vi "StripP(t).vi"(5 "d (depth of curvature)":dbl format="%.2f", 6 "strip (cm)":cluster{"radius":dbl, "h":dbl, "w":dbl}={"radius"=10.0, "h"=5.0, "w"=4.0} {"radius" format="%.2f"; "w" format="%.2f"; "h" format="%.2f"}, 7 "Ring":u16(ring) items=["Strip", "sphere section"], 8 "edge points":dbl[][](array[numeric]) format="%.2f", 9 "waveform sampling rate s":dbl=1e-08 format="%.2e", 10 "drive signal":dbl[](array[numeric])=[-0.5634920634920635, -0.6825396825396826, -0.8015873015873016, -0.9920634920634921, -1.1507936507936507, -1.3888888888888888, -1.992063492063492, -4.2063492063492065, -5.888888888888889, 13.023809523809524, 61.32539682539682, 92.83333333333333, 75.10317460317461, 18.126984126984127, -54.93650793650794, -109.60317460317461, -104.22222222222223, 18.134920634920636, 83.33333333333333, 27.27777777777778, -42.19047619047619, -45.63492063492063, 10.15079365079365, 49.05555555555556, 28.19047619047619, -5.658730158730159, -15.261904761904763, -4.4603174603174605, 7.984126984126984, 10.682539682539682, 5.809523809523809, -0.03968253968253968, -2.515873015873016, -1.4841269841269842, 1.0396825396825398, 2.0555555555555554, 0.9523809523809523, -0.6031746031746031, -1.007936507936508, -0.3968253968253968, 0.14285714285714285] format="%.2f", 11 "P (cm)":cluster{"x":dbl, "y":dbl, "z":dbl}={"x"=-4.0, "y"=0.0, "z"=4.0} {"x" format="%.2f"; "z" format="%.2f"; "y" format="%.2f"}) -> (2 "Waveform Graph":dbl[](graph), 3 "min time shift":dbl format="%.2f")   [LabVIEW 2022 SP3]
panel:
  out "In focal Zone?":bool
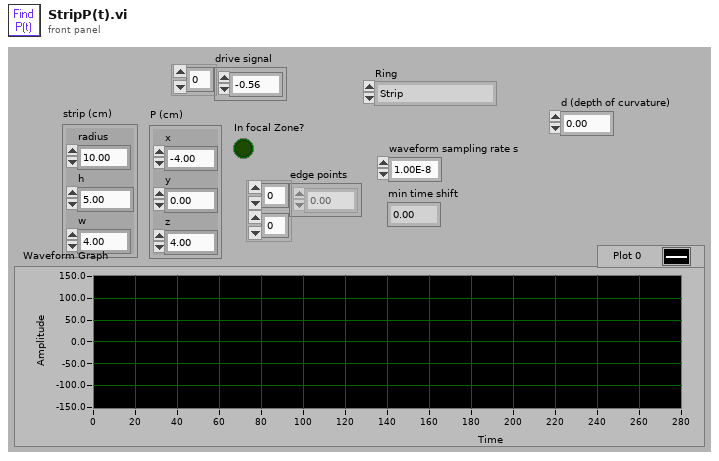
[diagram p1: front panel]
types:
  T1 = cluster{"r":dbl, "d":dbl, "c (cm/s)":dbl, "waveform sampling rate s":dbl, bool}
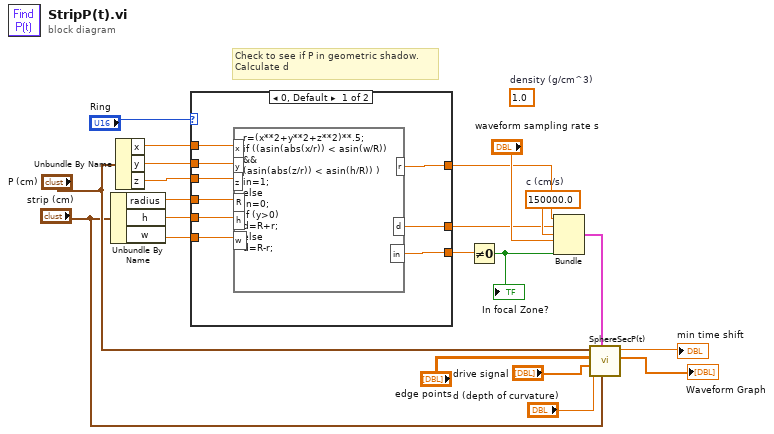
[diagram p0: block diagram]
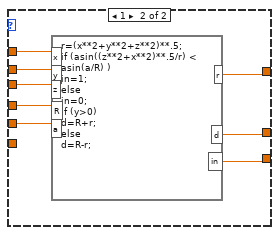
[diagram p2: hidden frame]
diagram:
  (unwired) 1.0  # density (g/cm^3)
  w21 = 150000.0  # c (cm/s)
  # "Check to see if P in geometric shadow.\nCalculate d"
  n1 = Unbundle By Name("strip (cm)") -> ("radius"=w6:dbl, "h"=w15:dbl, "w"=w14:dbl)
  n2 = Unbundle By Name("P (cm)") -> ("x"=w18:dbl, "y"=w17:dbl, "z"=w16:dbl)
  n3 = case shown="0, Default" "Ring" {
    tunnel: w18 -> [w30 w38]
    tunnel: w17 -> [w29 w37]
    tunnel: w16 -> [w28 w36]
    tunnel: w15 -> [w27 w34]
    tunnel: w14 -> [w26 _]
    tunnel: [w25 w31] -> w13
    tunnel: [w24 w32] -> w11
    tunnel: [w23 w33] -> w9
    tunnel: w6 -> [w22 w35]
    frame 0, Default {
      n4 = formula code="r=(x**2+y**2+z**2)**.5;\nif ((asin(abs(x/r)) < asin(w/R)) &&\n(asin(abs(z/r)) < asin(h/R)) )\nin=1;\nelse\nin=0;\nif (y>0)\nd=R+r;\nelse\nd=R-r;"("y"=w29, "x"=w30, "z"=w28, "R"=w22, "h"=w27, "w"=w26) -> ("in"=w25:dbl, "r"=w23:dbl, "d"=w24:dbl)
    }
    frame 1 {
      n5 = formula code="r=(x**2+y**2+z**2)**.5;\nif (asin((z**2+x**2)**.5/r) < asin(a/R) )\nin=1;\nelse\nin=0;\nif (y>0)\nd=R+r;\nelse\nd=R-r;"("y"=w37, "x"=w38, "z"=w36, "R"=w35, "a"=w34) -> ("in"=w31:dbl, "r"=w33:dbl, "d"=w32:dbl)
    }
  }
  n6 = Not Equal To 0?(x=w13) -> (x != 0?=w7:bool)
  "In focal Zone?" <- w7
  n7 = Bundle("r"=w9, "d"=w11, "c (cm/s)"=w21, "waveform sampling rate s"="waveform sampling rate s", w7) -> (w2:T1)  [unwired: 1 out]
  n8 = call "SphereSecP(t).vi"("strip (cm)"="strip (cm)", "Cluster"=w2, "d (depth of curvature)"="d (depth of curvature)", "Drive signal"="drive signal", "edge points"="edge points", "P (cm)"="P (cm)") -> ("Pressure Wave"=→"Waveform Graph":dbl[], "min time shift"=→"min time shift":dbl)  [unwired: 4 out]
